vi "GT Get Compensate.vi"(0 "cardNum":i16, 1 "axis":i16, 2 "pPitchError":dbl, 3 "pCrossError":dbl, 4 "pBacklashError":dbl, 5 "pEncPos":dbl, 6 "pPrfPos":dbl, 7 "error in (no error)":errorcluster caption="错误输入（无错误）") -> (20 "function return":i16, 22 "pPitchError out":dbl, 23 "pCrossError out":dbl, 24 "pBacklashError out":dbl, 25 "pEncPos out":dbl, 26 "pPrfPos out":dbl, 27 "error out":errorcluster caption="错误输出")   [LabVIEW 2020, in "gts.lvlib"]
doc: "GT_API GT_GetCompensate(short cardNum,short axis,double *pPitchError,double *pCrossError,double *pBacklashError,double *pEncPos,double *pPrfPos);"
uses:
  gts.lvlib
  dll/32bit/multi_card/gts.dll
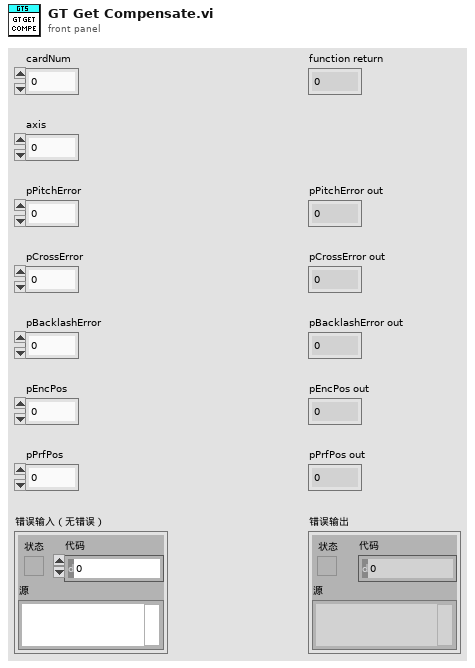
[diagram p1: front panel]
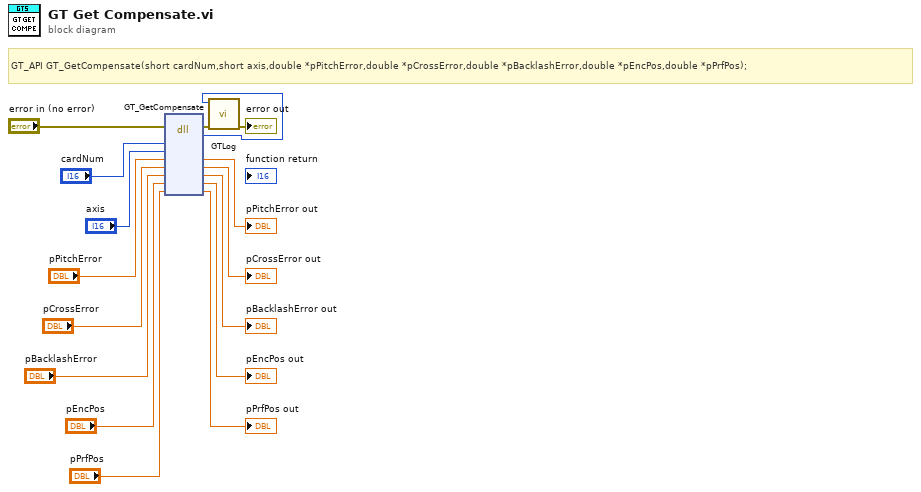
[diagram p0: block diagram]
diagram:
  # "GT_API GT_GetCompensate(short cardNum,short axis,double *pPitchError,double *pCrossError,double *pBacklashError,double *pEncPos,double *pPrfPos);"
  n1 = dll-call lib="C:/1228/dll/32bit/multi_card/gts.dll" fn="GT_GetCompensate"(error in="error in (no error)", "cardNum"="cardNum", "axis"="axis", "pPitchError"="pPitchError", "pCrossError"="pCrossError", "pBacklashError"="pBacklashError", "pEncPos"="pEncPos", "pPrfPos"="pPrfPos") -> (error out=w3:errorcluster, w1:i16, "pPitchError"=→"pPitchError out":dbl, "pCrossError"=→"pCrossError out":dbl, "pBacklashError"=→"pBacklashError out":dbl, "pEncPos"=→"pEncPos out":dbl, "pPrfPos"=→"pPrfPos out":dbl)  [unwired: 4 in, 1 out]
  n2 = call "GTLog.vi"("error in (no error)"=w3, "Numeric"=w1) -> ("error out"=→"error out":errorcluster)  [unwired: 9 in]
